vi "6-t-invdist.vi"(8 "error in":errorcluster caption="err in", 9 "R(t)":dbl, 10 "F(t)":dbl, 11 "p_LExp":T1) -> (0 "error out":errorcluster caption="err out", 2 "t":dbl, 3 "p_LExp":T1)   [LabVIEW 2010, in "lv_02.lvlib"]
uses:
  lv_02.lvlib
  p_5E6_Lexp.ctl
  p_5E7_LW.ctl
  7-t-invdist.vi
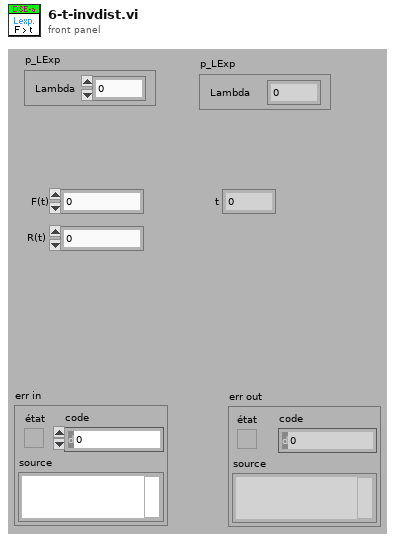
[diagram p1: front panel]
types:
  T1 = typedef "lv_02.lvlib/p_5E6_Lexp.ctl" = cluster{"Lambda":dbl}
  T2 = typedef "lv_02.lvlib/p_5E7_LW.ctl" = cluster{"Beta":dbl, "Eta":dbl, "Gama":dbl}
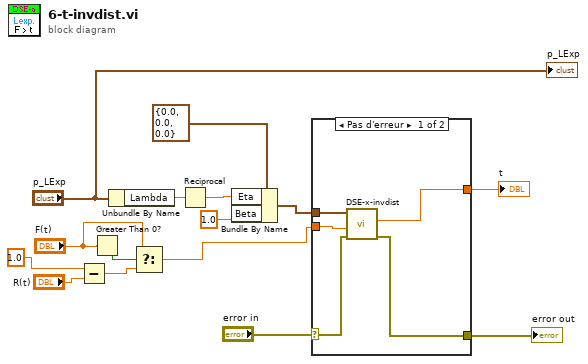
[diagram p0: block diagram]
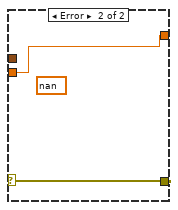
[diagram p2: hidden frame]
diagram:
  n1 = Subtract(x=1.0, y="R(t)") -> (x-y=w1:dbl)
  n2 = Greater Than 0?(x="F(t)") -> (x > 0?=w6:bool)
  n3 = Unbundle By Name("p_LExp") -> ("Lambda"=w11:dbl)
  n4 = Select(t="F(t)", s=w6, f=w1) -> (s? t:f=w4:dbl)
  n5 = Reciprocal(x=w11) -> (1/x=w10:dbl)
  n6 = Bundle By Name(cluster=T2 {"Beta"=0.0, "Eta"=0.0, "Gama"=0.0} ("p_LW"), "Eta"=w10, "Beta"=1.0) -> (w8:T2)
  n7 = case shown="Pas d'erreur" "error in" {
    selector: "error in" -> [w19 w22]
    tunnel: w4 -> [w16 w21]
    tunnel: [w18 w22] -> w14
    tunnel: w8 -> [w20 _]
    tunnel: [w17 w21] -> w7
    frame No Error {
      n8 = call-poly "DSE-x-invdist.vi"("error in"=w19, "R(t)"=w16, "p_LW"=w20) -> ("error out"=w18:errorcluster, "t"=w17:dbl)  [unwired: 6 in, 1 out]
    }
    frame Error {
      (unwired) nan
    }
  }
  "error out" <- w14
  "t" <- w7
  "p_LExp" <- "p_LExp"
